vi "parse-JSON.vi"(8 "JSON Structure (cluster)":T1, 11 "VISA resource name in":refnum<visa-resource-name>) -> (0 "pid":string, 1 "data":cluster{"engine":i32, "shaft":i32}, 2 "chksum":i32, 3 "VISA Refnum out":refnum<visa-resource-name>)   [LabVIEW 2013]
panel:
  out "String":string
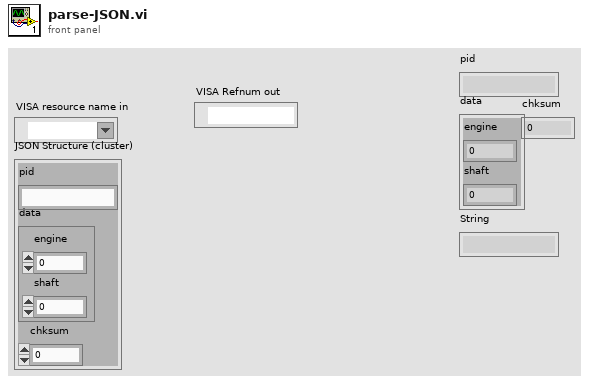
[diagram p1: front panel]
types:
  T1 = cluster{"pid":string, "data":cluster{"engine":i32, "shaft":i32}, "chksum":i32}
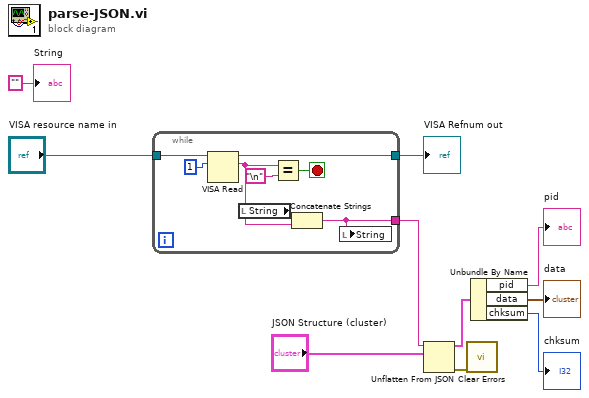
[diagram p0: block diagram]
diagram:
  n1 = while {
    tunnel: "VISA resource name in" -> [w18]
    tunnel: [w17] -> w10
    tunnel: [w11] -> w6
    stop <- w14 stop-if-true
    n2 = VISA Read(VISA resource name=w18, byte count=u32 1) -> (VISA resource name out=w17:refnum<visa-resource-name>, read buffer=w16:string)  [unwired: 1 in, 2 out]
    n3 = local read "String"() -> (w12:string)
    n4 = Equal?(x=w16, y="\n") -> (x = y?=w14:bool)
    n5 = Concatenate Strings(w12, w16) -> (w11:string)
    n6 = local write "String"(w11) -> ()
  }
  "VISA Refnum out" <- w10
  n7 = Unflatten From JSON(JSON string=w6, type and defaults="JSON Structure (cluster)") -> (value=w4:T1, error out=w7:errorcluster)  [unwired: 5 in]
  n8 = call <vilib>:"Clear Errors.vi"("error in (no error)"=w7) -> ()  [unwired: 6 in, 1 out]
  n9 = Unbundle By Name(w4) -> ("pid"=→"pid":string, "data"=→"data":cluster{"engine":i32, "shaft":i32}, "chksum"=→"chksum":i32)
  "String" <- ""
